vi "open_write.vi"   [LabVIEW 2016]
panel:
  # "CTRL-E (PC) or Command-E (Mac) to open the block diagram."
types:
  T1 = typedef "LVHSConnector.ctl" = refnum<class "BrickReference.lvclass">
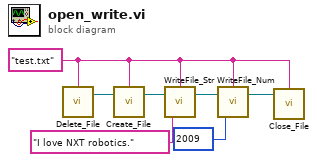
[diagram p0: block diagram]
diagram:
  w1 = "test.txt" ("Filename")
  n1 = call <vilib>:"Delete_File.vi"("Filename"=w1) -> ("NXT/EV3"=w7:T1)  [unwired: 3 in]
  n2 = call <vilib>:"Create_File.vi"("NXT/EV3"=w7, "Filename"=w1) -> ("NXT/EV3"=w6:T1)  [unwired: 2 in]
  n3 = call <vilib>:"WriteFile_Str.vi"("String"="I love NXT robotics.", "NXT/EV3"=w6, "Filename"=w1) -> ("NXT/EV3"=w4:T1)  [unwired: 1 in]
  n4 = call <vilib>:"WriteFile_Num.vi"("Number"=2009, "NXT/EV3"=w4, "Filename"=w1) -> ("NXT/EV3"=w3:T1)  [unwired: 1 in]
  n5 = call <vilib>:"Close_File.vi"("NXT/EV3"=w3, "Filename"=w1) -> ()  [unwired: 2 in, 1 out]
